vi "DSF.Engine.Builder.Set Thread Parameters.vi"(10 "Thread Parameters":refnum<class "Thread Parameters.lvclass">, 11 "Builder in":refnum<class "DSF.Engine.Builder.lvclass">) -> (3 "Builder out":refnum<class "DSF.Engine.Builder.lvclass">)   [LabVIEW 2016, in "DSF.Engine.lvlib" / "DSF.Engine.Builder.lvclass"]
uses:
  DSF.Engine.Builder.lvclass
  Thread Parameters/Thread Parameters.lvclass
  DSF.Engine.Builder.lvclass/DSF.Engine.Builder.ctl
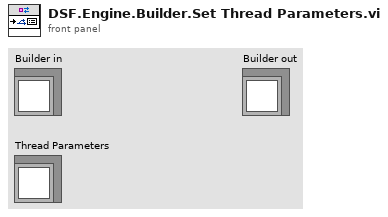
[diagram p1: front panel]
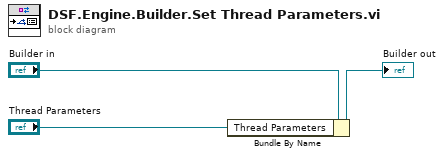
[diagram p0: block diagram]
diagram:
  n1 = Bundle By Name(cluster="Builder in", "Thread Parameters"="Thread Parameters") -> (→"Builder out":refnum<class "DSF.Engine.Builder.lvclass">)
